vi "SweepRangeToList.vi"(11 "sweep ranges":T1(array[cluster])) -> (1 "totalNumberOfPoints":i32, 3 "sweep freq list":cluster{"frequency":dbl, "bandwidth":dbl}[](array[cluster]))   [LabVIEW 2017, in "EmsaAcquisition.lvlib"]
uses:
  <vilib>/addons/InsightCM/Devices/Shared/Emsa/EmsaAcquisition/EmsaAcquisition.lvlib
  <vilib>/Analysis/1siggen.llb/Ramp Pattern by Samples.vi
  <vilib>/Analysis/NI_AALBase.lvlib
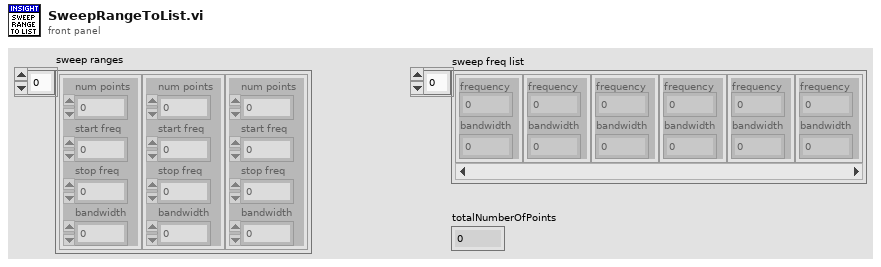
[diagram p1: front panel]
types:
  T1 = cluster{"num points":i32, "start freq":dbl, "stop freq":dbl, "bandwidth":dbl}[]
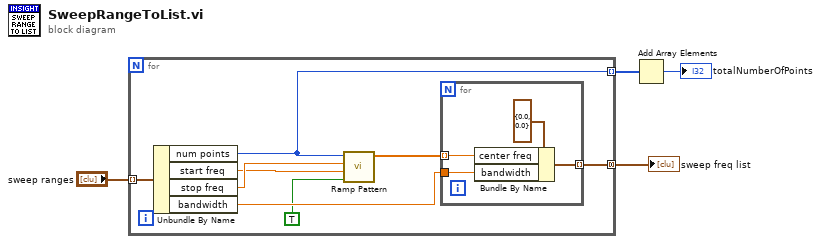
[diagram p0: block diagram]
diagram:
  n1 = for {
    tunnel: "sweep ranges" -> [w12] mode=indexing
    tunnel: [w7] -> w3 mode=concatenating
    tunnel: [w5] -> w2 mode=indexing
    n2 = Unbundle By Name(w12) -> ("num points"=w5:i32, "start freq"=w10:dbl, "stop freq"=w11:dbl, "bandwidth"=w8:dbl)
    n3 = call-poly <vilib>:"Ramp Pattern.vi"("exclude end?"=TRUE, "start"=w10, "end"=w11, "samples"=w5) -> ("Ramp Pattern"=w9:dbl[])  [unwired: 6 in, 1 out]
    n4 = for {
      tunnel: w9 -> [w15] mode=indexing
      tunnel: w8 -> [w14]
      tunnel: [w13] -> w7 mode=indexing
      n5 = Bundle By Name(cluster=cluster{"center freq":dbl, "bandwidth":dbl} {"center freq"=0.0, "bandwidth"=0.0} ("frequency band"), "center freq"=w15, "bandwidth"=w14) -> (w13:cluster{"center freq":dbl, "bandwidth":dbl})
    }
  }
  "sweep freq list" <- w3
  n6 = Add Array Elements(numeric array=w2) -> (sum=→"totalNumberOfPoints":i32)
